vi "ConversionScaleFactor.vi"(9 "Desired Unit":string, 10 "Original Unit":string, 11 "Conversion Op":T1) -> (3 "Scale Factor":dbl)   [LabVIEW 2017, in "CmsVirtualChannel.lvlib"]
uses:
  <vilib>/addons/InsightCM/Devices/Shared/Cms/CmsVirtualChannel/CmsVirtualChannel.lvlib
  <vilib>/addons/InsightCM/Utilities/Analysis/Shared/controls/ConversionOp.ctl
  <vilib>/addons/_NISVFA/_Shared subVIs/Controls/svc_Engineering Units Text Ring.ctl
  <vilib>/addons/InsightCM/Utilities/Analysis/Shared/AnalysisHelper.lvlib
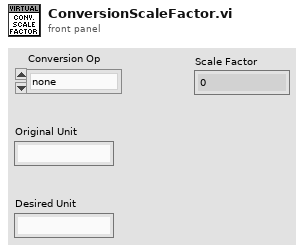
[diagram p1: front panel]
types:
  T1 = typedef "AnalysisHelper.lvlib/ConversionOp.ctl" = enum16{"none", "singleInt", "doubleInt", "singleDiff", "doubleDiff"}
  T2 = enum16{"single integration", "double integration", "single differentiation", "double differentiation", "none"}
  T3 = typedef "svc_Engineering Units Text Ring.ctl" = u16
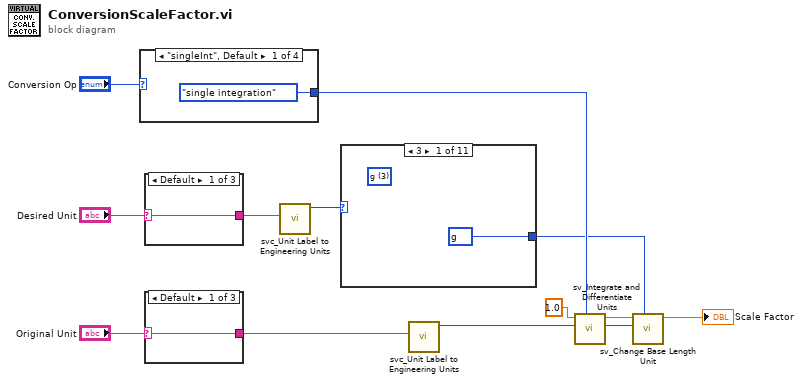
[diagram p0: block diagram]
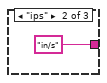
[diagram p2: hidden frame]
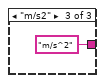
[diagram p3: hidden frame]
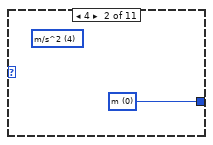
[diagram p4: hidden frame]
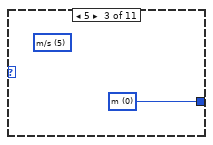
[diagram p5: hidden frame]
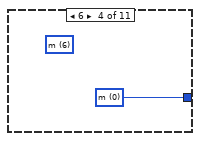
[diagram p6: hidden frame]
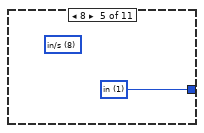
[diagram p7: hidden frame]
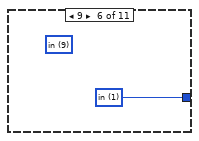
[diagram p8: hidden frame]
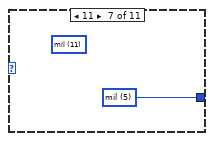
[diagram p9: hidden frame]
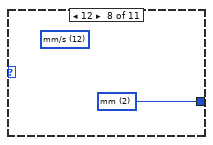
[diagram p10: hidden frame]
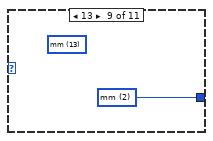
[diagram p11: hidden frame]
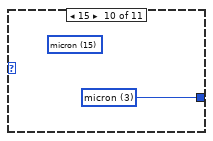
[diagram p12: hidden frame]
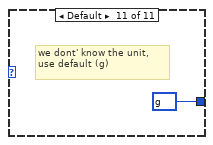
[diagram p13: hidden frame]
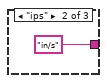
[diagram p14: hidden frame]
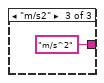
[diagram p15: hidden frame]
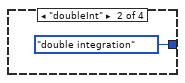
[diagram p16: hidden frame]
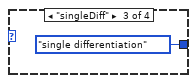
[diagram p17: hidden frame]
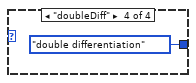
[diagram p18: hidden frame]
diagram:
  n1 = case shown="\"singleInt\", Default" "Conversion Op" {
    tunnel: [T2."single integration" ("Integration Type") T2."double integration" ("Integration Type") T2."single differentiation" ("Integration Type") T2."double differentiation" ("Integration Type")] -> w11
    frame "singleInt", Default {
    }
    frame "doubleInt" {
    }
    frame "singleDiff" {
    }
    frame "doubleDiff" {
    }
  }
  n2 = case shown="Default" "Desired Unit" {
    selector: "Desired Unit" -> [w18 _ _]
    tunnel: [w18 "in/s" "m/s^2"] -> w13
    frame Default {
    }
    frame "ips" {
    }
    frame "m/s2" {
    }
  }
  n3 = case shown="Default" "Original Unit" {
    selector: "Original Unit" -> [w21 _ _]
    tunnel: [w21 "in/s" "m/s^2"] -> w1
    frame Default {
    }
    frame "ips" {
    }
    frame "m/s2" {
    }
  }
  n4 = call <vilib>:"svc_Unit Label to Engineering Units.vi"("unit label"=w13) -> ("engineering units"=w7:T3)  [unwired: 9 in, 1 out]
  n5 = case shown="3" w7 {
    tunnel: [w24 w25 w26 w27 w28 w29 w30 w31 w32 w33 w34] -> w6
    frame 3 {
      w24 = 386 items=["no change"=-1, "g"=386, "m"=0, "cm"=4, "mm"=2, "micron"=3, "in"=1, "mil"=5] ("desired base units for vibration")
      (unwired) T3 3 items=["custom..."=0, "V"=1, "A"=21, "Pa"=2, "N"=20, "g"=3, "m/s^2"=4, "m/s"=5, "m"=6, "mm/s"=12, "mm"=13, "micron/s"=14, "micron"=15, "in/s^2"=7, "in/s"=8, "in"=9, "mil/s"=10, "mil"=11, "rad/s^2"=16, "rad/s"=17, "rad"=18, "deg/s^2"=26, "deg/s"=27, "deg"=28, "RPM"=22, "cycle/s^2"=23, "Hz"=24, "cycle"=25, "strain"=19] ("engineering units")
    }
    frame 4 {
      w25 = 0 items=["no change"=-1, "g"=386, "m"=0, "cm"=4, "mm"=2, "micron"=3, "in"=1, "mil"=5] ("desired base units for vibration")
      (unwired) T3 4 items=["custom..."=0, "V"=1, "A"=21, "Pa"=2, "N"=20, "g"=3, "m/s^2"=4, "m/s"=5, "m"=6, "mm/s"=12, "mm"=13, "micron/s"=14, "micron"=15, "in/s^2"=7, "in/s"=8, "in"=9, "mil/s"=10, "mil"=11, "rad/s^2"=16, "rad/s"=17, "rad"=18, "deg/s^2"=26, "deg/s"=27, "deg"=28, "RPM"=22, "cycle/s^2"=23, "Hz"=24, "cycle"=25, "strain"=19] ("engineering units")
    }
    frame 5 {
      w26 = 0 items=["no change"=-1, "g"=386, "m"=0, "cm"=4, "mm"=2, "micron"=3, "in"=1, "mil"=5] ("desired base units for vibration")
      (unwired) T3 5 items=["custom..."=0, "V"=1, "A"=21, "Pa"=2, "N"=20, "g"=3, "m/s^2"=4, "m/s"=5, "m"=6, "mm/s"=12, "mm"=13, "micron/s"=14, "micron"=15, "in/s^2"=7, "in/s"=8, "in"=9, "mil/s"=10, "mil"=11, "rad/s^2"=16, "rad/s"=17, "rad"=18, "deg/s^2"=26, "deg/s"=27, "deg"=28, "RPM"=22, "cycle/s^2"=23, "Hz"=24, "cycle"=25, "strain"=19] ("engineering units")
    }
    frame 6 {
      w27 = 0 items=["no change"=-1, "g"=386, "m"=0, "cm"=4, "mm"=2, "micron"=3, "in"=1, "mil"=5] ("desired base units for vibration")
      (unwired) T3 6 items=["custom..."=0, "V"=1, "A"=21, "Pa"=2, "N"=20, "g"=3, "m/s^2"=4, "m/s"=5, "m"=6, "mm/s"=12, "mm"=13, "micron/s"=14, "micron"=15, "in/s^2"=7, "in/s"=8, "in"=9, "mil/s"=10, "mil"=11, "rad/s^2"=16, "rad/s"=17, "rad"=18, "deg/s^2"=26, "deg/s"=27, "deg"=28, "RPM"=22, "cycle/s^2"=23, "Hz"=24, "cycle"=25, "strain"=19] ("engineering units")
    }
    frame 8 {
      w28 = 1 items=["no change"=-1, "g"=386, "m"=0, "cm"=4, "mm"=2, "micron"=3, "in"=1, "mil"=5] ("desired base units for vibration")
      (unwired) T3 8 items=["custom..."=0, "V"=1, "A"=21, "Pa"=2, "N"=20, "g"=3, "m/s^2"=4, "m/s"=5, "m"=6, "mm/s"=12, "mm"=13, "micron/s"=14, "micron"=15, "in/s^2"=7, "in/s"=8, "in"=9, "mil/s"=10, "mil"=11, "rad/s^2"=16, "rad/s"=17, "rad"=18, "deg/s^2"=26, "deg/s"=27, "deg"=28, "RPM"=22, "cycle/s^2"=23, "Hz"=24, "cycle"=25, "strain"=19] ("engineering units")
    }
    frame 9 {
      w29 = 1 items=["no change"=-1, "g"=386, "m"=0, "cm"=4, "mm"=2, "micron"=3, "in"=1, "mil"=5] ("desired base units for vibration")
      (unwired) T3 9 items=["custom..."=0, "V"=1, "A"=21, "Pa"=2, "N"=20, "g"=3, "m/s^2"=4, "m/s"=5, "m"=6, "mm/s"=12, "mm"=13, "micron/s"=14, "micron"=15, "in/s^2"=7, "in/s"=8, "in"=9, "mil/s"=10, "mil"=11, "rad/s^2"=16, "rad/s"=17, "rad"=18, "deg/s^2"=26, "deg/s"=27, "deg"=28, "RPM"=22, "cycle/s^2"=23, "Hz"=24, "cycle"=25, "strain"=19] ("engineering units")
    }
    frame 11 {
      w30 = 5 items=["no change"=-1, "g"=386, "m"=0, "cm"=4, "mm"=2, "micron"=3, "in"=1, "mil"=5] ("desired base units for vibration")
      (unwired) T3 11 items=["custom..."=0, "V"=1, "A"=21, "Pa"=2, "N"=20, "g"=3, "m/s^2"=4, "m/s"=5, "m"=6, "mm/s"=12, "mm"=13, "micron/s"=14, "micron"=15, "in/s^2"=7, "in/s"=8, "in"=9, "mil/s"=10, "mil"=11, "rad/s^2"=16, "rad/s"=17, "rad"=18, "deg/s^2"=26, "deg/s"=27, "deg"=28, "RPM"=22, "cycle/s^2"=23, "Hz"=24, "cycle"=25, "strain"=19] ("engineering units")
    }
    frame 12 {
      w31 = 2 items=["no change"=-1, "g"=386, "m"=0, "cm"=4, "mm"=2, "micron"=3, "in"=1, "mil"=5] ("desired base units for vibration")
      (unwired) T3 12 items=["custom..."=0, "V"=1, "A"=21, "Pa"=2, "N"=20, "g"=3, "m/s^2"=4, "m/s"=5, "m"=6, "mm/s"=12, "mm"=13, "micron/s"=14, "micron"=15, "in/s^2"=7, "in/s"=8, "in"=9, "mil/s"=10, "mil"=11, "rad/s^2"=16, "rad/s"=17, "rad"=18, "deg/s^2"=26, "deg/s"=27, "deg"=28, "RPM"=22, "cycle/s^2"=23, "Hz"=24, "cycle"=25, "strain"=19] ("engineering units")
    }
    frame 13 {
      w32 = 2 items=["no change"=-1, "g"=386, "m"=0, "cm"=4, "mm"=2, "micron"=3, "in"=1, "mil"=5] ("desired base units for vibration")
      (unwired) T3 13 items=["custom..."=0, "V"=1, "A"=21, "Pa"=2, "N"=20, "g"=3, "m/s^2"=4, "m/s"=5, "m"=6, "mm/s"=12, "mm"=13, "micron/s"=14, "micron"=15, "in/s^2"=7, "in/s"=8, "in"=9, "mil/s"=10, "mil"=11, "rad/s^2"=16, "rad/s"=17, "rad"=18, "deg/s^2"=26, "deg/s"=27, "deg"=28, "RPM"=22, "cycle/s^2"=23, "Hz"=24, "cycle"=25, "strain"=19] ("engineering units")
    }
    frame 15 {
      w33 = 3 items=["no change"=-1, "g"=386, "m"=0, "cm"=4, "mm"=2, "micron"=3, "in"=1, "mil"=5] ("desired base units for vibration")
      (unwired) T3 15 items=["custom..."=0, "V"=1, "A"=21, "Pa"=2, "N"=20, "g"=3, "m/s^2"=4, "m/s"=5, "m"=6, "mm/s"=12, "mm"=13, "micron/s"=14, "micron"=15, "in/s^2"=7, "in/s"=8, "in"=9, "mil/s"=10, "mil"=11, "rad/s^2"=16, "rad/s"=17, "rad"=18, "deg/s^2"=26, "deg/s"=27, "deg"=28, "RPM"=22, "cycle/s^2"=23, "Hz"=24, "cycle"=25, "strain"=19] ("engineering units")
    }
    frame Default {
      w34 = 386 items=["no change"=-1, "g"=386, "m"=0, "cm"=4, "mm"=2, "micron"=3, "in"=1, "mil"=5] ("desired base units for vibration")
      # "we dont' know the unit,\nuse default (g)"
    }
  }
  n6 = call <vilib>:"svc_Unit Label to Engineering Units.vi"("unit label"=w1) -> ("engineering units"=w10:T3)  [unwired: 9 in, 1 out]
  n7 = call <vilib>:"sv_Integrate and Differentiate Units.vi"("integration type"=w11, "engineering units in"=w10, "input value"=1.0) -> ("engineering units out"=w8:T3, "output value"=w9:dbl)  [unwired: 4 in, 1 out]
  n8 = call <vilib>:"sv_Change Base Length Unit.vi"("desired base units for vibration"=w6, "engineering units in"=w8, "value in [EU]"=w9) -> ("value out [desired EU]"=→"Scale Factor":dbl)  [unwired: 4 in, 2 out]
